vi "twice.vi"(1 "x":i16) -> (0 "y":i16)   [LabVIEW 2018, in "posit.lvlib"]
uses:
  posit.lvlib
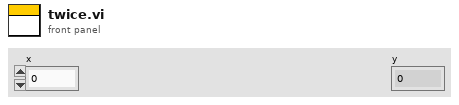
[diagram p1: front panel]
types:
  T1 = typedef "posit.lvlib/unpacked.ctl" = cluster{"sign":bool, "regime":i16, "exoinent":i16, "fraction":i16, "type":T2}
  T2 = typedef "posit.lvlib/specialnumber.ctl" = enum16{"Zero", "Regular", "NaN", "Infinity"}
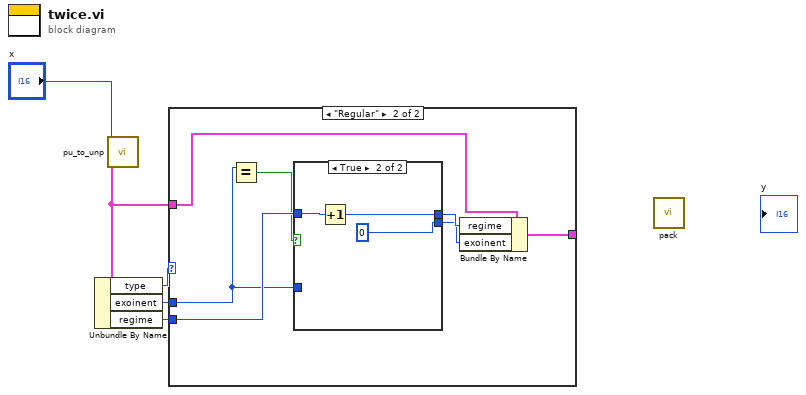
[diagram p0: block diagram]
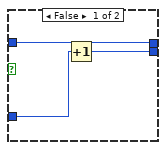
[diagram p3: hidden frame]
diagram:
  n1 = call "pu_to_unp.vi"("x"="x") -> ("y"=w1:T1)  [unwired: 10 in]
  n2 = Unbundle By Name(w1) -> ("type"=w4:T2, "exoinent"=w3:i16, "regime"=w2:i16)
  n3 = case shown="\"Regular\"" w4 {
    tunnel: w3 -> [_ w12]
    tunnel: w2 -> [_ w13]
    tunnel: w1 -> [w6 w11]
    tunnel: [w6 w10] -> _
    frame "Zero", Default {
    }
    frame "Regular" {
      n4 = Equal?(x=w12) -> (x = y?=w7:bool)  [unwired: 1 in]
      n5 = case shown="True" w7 {
        tunnel: w13 -> [w14 w19]
        tunnel: w12 -> [w16 _]
        tunnel: [w15 i16 0] -> w8
        tunnel: [w14 w18] -> w9
        frame False {
          n6 = Increment(x=w16) -> (x+1=w15:i16)
        }
        frame True {
          n7 = Increment(x=w19) -> (x+1=w18:i16)
        }
      }
      n8 = Bundle By Name(cluster=w11, "regime"=w9, "exoinent"=w8) -> (w10:T1)
    }
  }
  n9 = call "pack.vi"() -> ()  [unwired: 12 in]
